vi "GPIB_autodetect.vi"(8 "error in (no error)":errorcluster, 9 "Verify GPIB address":bool, 10 "Instrument GPIB address in":string, 11 "InstrControl in":refnum<class "InstrControl.lvclass">) -> (0 "error out":errorcluster, 2 "Instrument GPIB address":string, 3 "InstrControl out":refnum<class "InstrControl.lvclass">)   [LabVIEW 2018, in "InstrControl.lvclass"]
uses:
  InstrControl.lvclass
panel:
  out "instrument responses":string[](array[string])
  out "GPIB addresses found":string[](array[string])
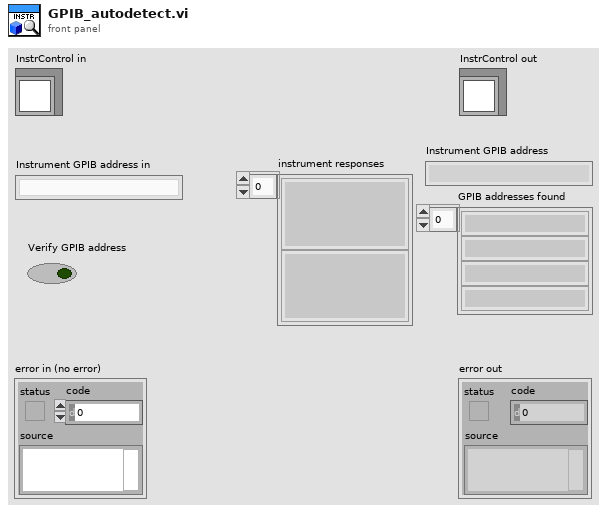
[diagram p1: front panel]
types:
  T1 = cluster{"error":bool, "code":i32, "source":string}
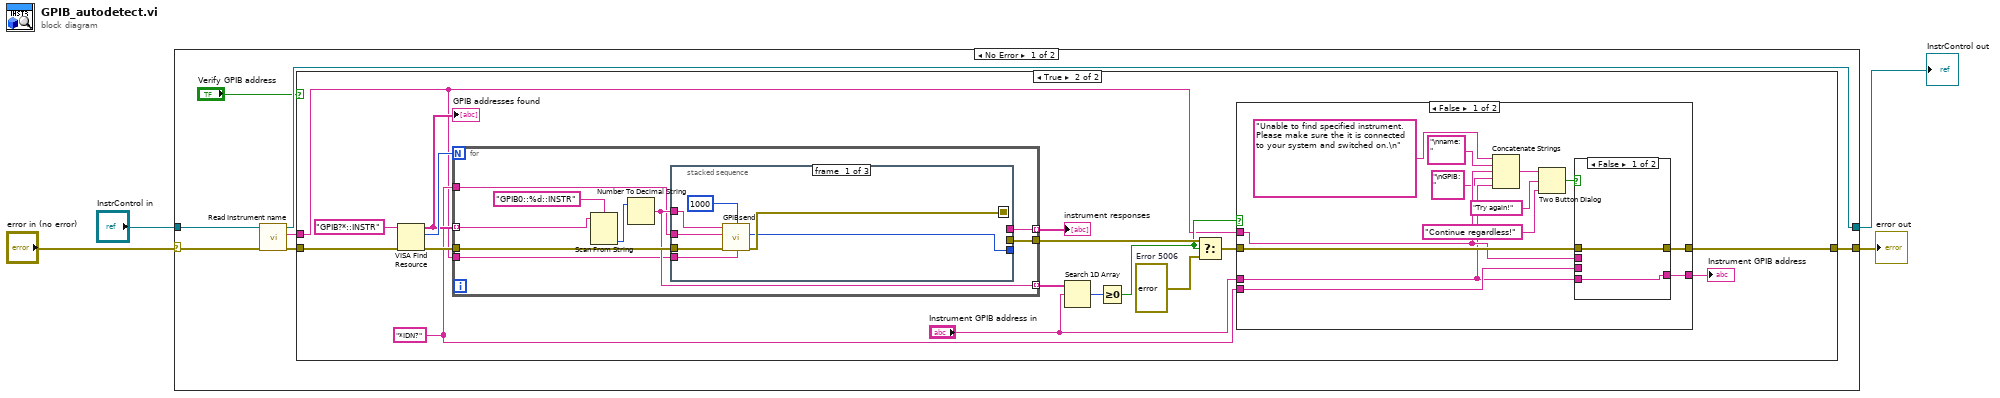
[diagram p0: block diagram]
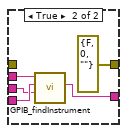
[diagram p3: hidden frame]
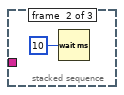
[diagram p5: hidden frame]
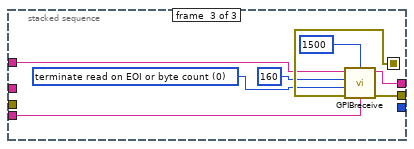
[diagram p6: hidden frame]
diagram:
  n1 = case shown="No Error" "error in (no error)" {
    selector: "error in (no error)" -> [w10 w78]
    tunnel: [w7 w78] -> w3
    tunnel: [w9 w77] -> w1
    tunnel: "InstrControl in" -> [w11 w77]
    frame No Error {
      n2 = call-dynamic "Read Instrument name.vi"("error in (no error)"=w10, "InstControl in"=w11) -> ("error out"=w8:errorcluster, "Instrument name"=w6:string, "InstControl out"=w9:refnum<class "InstrControl.lvclass">)  [unwired: 7 in]
      n3 = case shown="True" "Verify GPIB address" {
        tunnel: w8 -> [w12 w23]
        tunnel: [w12 w15] -> w7
        tunnel: w6 -> [_ w13]
        frame False {
        }
        frame True {
          w14 = "*IDN?" ("regular expression")
          w28 = errorcluster {"status"=FALSE, "code"=5005, "source"="Unable to find specified instrument.  Please make sure the it is connected to your system and switched on."}  # Error 5006
          n4 = VISA Find Resource(8:w23, 11:"GPIB?*::INSTR" ("expression (\"\")")) -> (0:w27:errorcluster, 2:w26:u32, 3:w25:string[])  [unwired: 1 in]
          "GPIB addresses found" <- w25
          n5 = for {
            N: w26 -> [_]
            tunnel: w25 -> [w58] mode=indexing
            tunnel: w27 -> [w60]
            tunnel: [w59] -> w29
            tunnel: [w54] -> w20 mode=indexing
            tunnel: w13 -> [w53]
            tunnel: [w55] -> w24 mode=indexing
            tunnel: w14 -> [w52]
            n6 = Scan From String(format string="GPIB0::%d::INSTR" ("expression (\"\")"), input string=w58) -> (output 1=w56:i32)  [unwired: 3 in, 3 out]
            n7 = Number To Decimal String(number=w56) -> (decimal integer string=w54:string)  [unwired: 1 in]
            n8 = stacked-sequence {
              seq-local: [w65 _ _] -> [_ _ w75]
              tunnel: w54 -> [w67 _ w74]
              tunnel: w60 -> [w66 _ _]
              tunnel: [_ _ w76] -> w59
              tunnel: [_ _ w71] -> w55
              tunnel: w53 -> [w63 _ w72]
              tunnel: w52 -> [w62 _ _]
              tunnel: [w61 _ _] -> _
              frame #0 {
                n9 = call "GPIBsend.vi"("timeout ms"=u32 1000, "address string"=w67, "write buffer"=w62, "source"=w63, "error in"=w66) -> ("byte count"=w61:i32, "error out"=w65:errorcluster)  [unwired: 2 in, 1 out]
              }
              frame #1 {
                n10 = Wait (ms)(milliseconds to wait=10) -> ()  [unwired: 1 out]
              }
              frame #2 {
                w70 = 0 items=["terminate read on EOI or byte count", "terminate read on EOI, byte count, or CR", "terminate read on EOI, byte count, or LF"] ("read mode")
                n11 = call "GPIBreceive.vi"("timeout ms"=u32 1500, "address string"=w74, "byte count"=160, "source"=w72, "read mode"=w70, "error in"=w75) -> ("read buffer"=w71:string, "error out"=w76:T1)  [unwired: 1 in, 1 out]
              }
            }
          }
          "instrument responses" <- w24
          n12 = Search 1D Array(1D array=w20, element="Instrument GPIB address in") -> (index of element=w19:i32)  [unwired: 1 in]
          n13 = Greater Or Equal To 0?(x=w19) -> (x >= 0?=w18:bool)
          n14 = Select(t=w29, s=w18, f=w28) -> (s? t:f=w16:errorcluster)
          n15 = case shown="False" w18 {
            tunnel: "Instrument GPIB address in" -> [w30 w51]
            tunnel: [w39 w51] -> w21
            tunnel: w16 -> [w38 w50]
            tunnel: [w37 w50] -> w15
            tunnel: w14 -> [w36 _]
            tunnel: w13 -> [w33 _]
            frame False {
              n16 = Concatenate Strings("Unable to find specified instrument.  Please make sure the it is connected to your system and switched on.\n" ("source"), "\nname: " ("string"), w33, "\nGPIB: " ("string"), w30) -> (w32:string)
              n17 = Two Button Dialog(message=w32, 1:"Continue regardless!", 2:"Try again!") -> (T button?=w40:bool)
              n18 = case shown="False" w40 {
                tunnel: w30 -> [w44 w49]
                tunnel: [w44 w48] -> w39
                tunnel: w38 -> [w43 _]
                tunnel: [w43 errorcluster {"status"=FALSE, "code"=0, "source"=""} ("error constant")] -> w37
                tunnel: w36 -> [_ w46]
                tunnel: w33 -> [_ w45]
                frame False {
                }
                frame True {
                  n19 = call "GPIB_findInstrument.vi"("ID command"=w46, "revised GPIB address"=w49, "Instrument name IN"=w45) -> ("revised GPIB address OUT"=w48:string)  [unwired: 8 in]
                }
              }
            }
            frame True {
            }
          }
          "Instrument GPIB address" <- w21
        }
      }
    }
    frame Error {
    }
  }
  "error out" <- w3
  "InstrControl out" <- w1
